vi "InverseKinematics.vi"(6 "L1":dbl, 9 "L2":dbl, 10 "y":dbl, 11 "x":dbl) -> (2 "theta1":dbl, 3 "theta2":dbl)   [LabVIEW 2024]
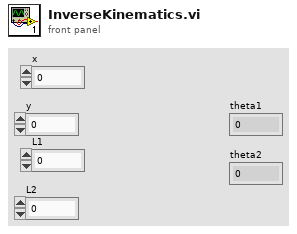
[diagram p1: front panel]
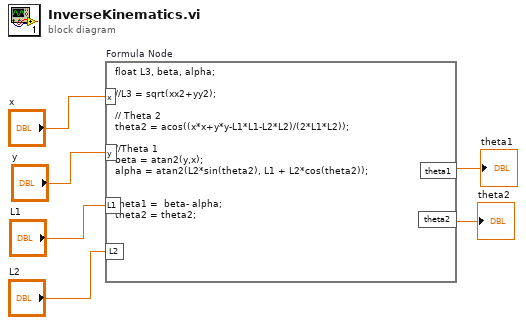
[diagram p0: block diagram]
diagram:
  n1 = formula code="float L3, beta, alpha;\n\n//L3 = sqrt(xx2+yy2);\n\n// Theta 2\ntheta2 = acos((x*x+y*y-L1*L1-L2*L2)/(2*L1*L2));\n\n//Theta 1\nbeta = atan2(y,x);\nalpha = atan2(L2*sin(theta2), L1 + L2*cos(theta2));\n\n\ntheta1 =  beta- alpha;\ntheta2 = theta2;"("L1"="L1", "L2"="L2", "x"="x", "y"="y") -> ("theta1"=→"theta1":dbl, "theta2"=→"theta2":dbl)
